vi "GetSiblings.vi"(8 "error in":errorcluster, 11 "node in":T1) -> (0 "error out":errorcluster, 3 "siblings":T1[](array[typedef]))   [LabVIEW 2013, in "NISE_CEF_Node.lvclass"]
uses:
  NISE_CEF_Node.lvclass
  NodeRef.ctl
  NISE_CEF_Node.lvclass/NISE_CEF_Node.ctl
  ReadParent.vi
  ReadChildren.vi
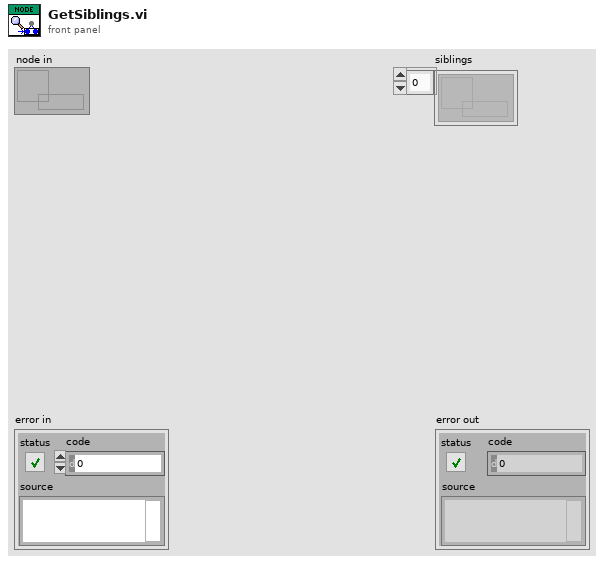
[diagram p1: front panel]
types:
  T1 = typedef "NISE_CEF_Node.lvclass/NodeRef.ctl" = refnum<data-value>
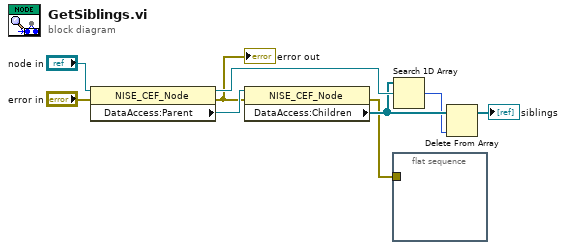
[diagram p0: block diagram]
diagram:
  n1 = property class="NISE_CEF_Node"(reference="node in", error in="error in") -> (reference out=w6:T1, error out=w1:errorcluster, "DataAccess:Parent"=w7:T1)
  "error out" <- w1
  n2 = property class="NISE_CEF_Node"(reference=w7, error in=w1) -> (error out=w2:errorcluster, "DataAccess:Children"=w5:T1[])  [unwired: 1 out]
  n3 = flat-sequence {
    tunnel: w2 -> [_]
    frame #0 {
    }
  }
  n4 = Search 1D Array(1D array=w5, element=w6) -> (index of element=w3:i32)  [unwired: 1 in]
  n5 = Delete From Array(array=w5, index=w3) -> (array with subset deleted=→"siblings":T1[])  [unwired: 1 in, 1 out]
